vi "ConfigureIOReference.vi"(8 "error in (no error)":errorcluster, 11 "Hardware Channel":string) -> (0 "error out":errorcluster, 1 "Model":u32, 2 "Channel Number":i32, 3 "IO Ref":refnum<k21>)   [LabVIEW 2017, in "ScanEngine.lvlib"]
uses:
  <vilib>/addons/InsightCM/Devices/Shared/Common/ScanEngine/ScanEngine.lvlib
  <resource>/objmgr/cRIO.rc
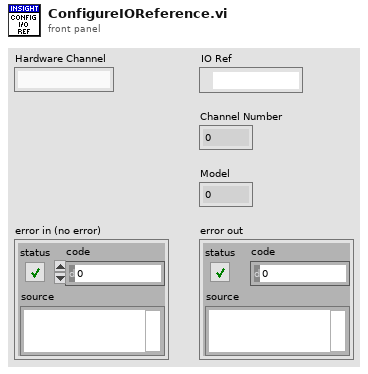
[diagram p1: front panel]
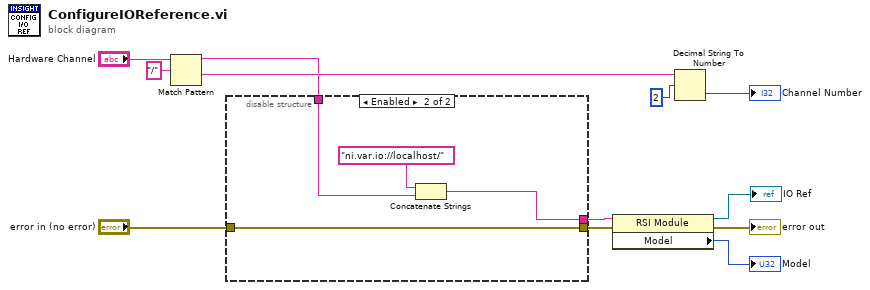
[diagram p0: block diagram]
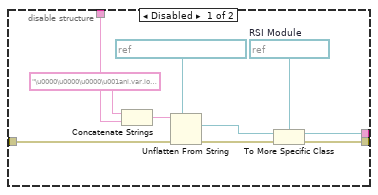
[diagram p2: hidden frame]
diagram:
  n1 = Match Pattern(string="Hardware Channel", regular expression="/") -> (before substring=w4:string, after substring=w7:string)  [unwired: 1 in, 2 out]
  n2 = disable-structure shown="Enabled" {
    disable-tunnel: [w22 w26] -> w12
    disable-tunnel: w4 -> [w19 w24]
    disable-tunnel: [w14 w23] -> w2
    disable-tunnel: "error in (no error)" -> [w13 w26]
    frame Disabled {
      w17 = refnum<k21> refnum  # RSI Module
      n3 = Concatenate Strings("\u0000\u0000\u0000\u001ani.var.io://localhost/" ("data string"), w19) -> (w18:string)
      n4 = Unflatten From String(type=refnum<k21> "ni.var.io://localhost" ("IO variable"), binary string=w18, error in (no error)=w13) -> (value=w16:refnum<k21>, error out=w15:errorcluster)  [unwired: 2 in, 1 out]
      n5 = To More Specific Class(target class=w17, reference=w16, error in=w15) -> (specific class reference=w14:refnum<k21>, error out=w22:errorcluster)
    }
    frame Enabled {
      n6 = Concatenate Strings("ni.var.io://localhost/" ("data string"), w24) -> (w23:string)
    }
  }
  n7 = property class="RSI Module"(reference=w2, error in=w12) -> (reference out=→"IO Ref":refnum<k21>, error out=→"error out":errorcluster, "Model"=→"Model":u32)
  n8 = Decimal String To Number(string=w7, offset=2 ("offset (0)")) -> (number=→"Channel Number":i32)  [unwired: 1 in, 1 out]
